vi "Frame Sample FIFO Experimental VI.vi"(8 "error in (no error)":errorcluster, 9 "reset in":bool, 10 "Hardware Configuration in":T1={"XY Stage"={"COM port"="", "XY stage available"=FALSE, "Baudrate"=0, "Type"=""}, "DAQ FPGA"={"Target"="RIO0", "input card type"=enum."AC Card", "Ref"=refnum, "Clock Freq (MHz) "=200.0, "Samples Wait after Trigger"=5080, "AOD fill"=4900, "StartupDelay"=0, "Slip Cycle (clock cycles)"=600000, "Add Cycle"=TRUE}, "Control system"={"Contrl Sys Available Ind"=FALSE, "Control system.FPGA Type"=enum."Virtex 7", "Control system.Network adapter name"="", "Control system.MAC address"="", "Control system.Ethernet Port"=0, "Ethernet opened"=FALSE, "Ctrl FPGA Clock (MHz)"=240.0, "AOD 1 Amplitude"=0, "AOD 2 Amplitude"=0, "AOD 3 Amplitude"=0, "AOD 4 Amplitude"=0, "AOD 5 Amplitude"=0, "AOD 6 Amplitude"=0, "Data Time Interval (ns)"=0.0, "T0 (ns)"=0.0, "Ta (ns)"=0.0}, "Encoder"={"IP address"="224.0.1.103", "Port"=7000, "Wheel radius (cm)"=16.0, "Encoder Trigger"=""}, "DAQmx Chan"={"Pockels AO"="", "Hard shutter AO"="", "PMT AOs"="", "Galvo AOs"="", "Power meter AI"=""}, "Computer MAC address"="", "Cam VidRec"={"DO flag-Video record"="", "DO flag-Trial start"=""}, "Externalise Triggers"=FALSE, "MC Supported"=FALSE, "Laser wavelength (nm)"=920.0} {"Laser wavelength (nm)" min=800.0 max=1080.0 step=1.0; "Encoder"."Wheel radius (cm)" format="%#_13g"; "Control system"."Control system.Ethernet Port" min=0 max=2048 step=1; "Control system"."Ctrl FPGA Clock (MHz)" min=80.0 max=500.0 step=1.0; "Control system"."Data Time Interval (ns)" min=0.0 max=2048.0 step=1.0; "Control system"."Ta (ns)" min=0.0 max=2048.0 step=1.0; "Control system"."T0 (ns)" min=0.0 max=2048.0 step=1.0; "Control system"."AOD 6 Amplitude" min=0 max=2048 step=1; "Control system"."AOD 5 Amplitude" min=0 max=2048 step=1; "Control system"."AOD 4 Amplitude" min=0 max=2048 step=1; "Control system"."AOD 3 Amplitude" min=0 max=2048 step=1; "Control system"."AOD 2 Amplitude" min=0 max=2048 step=1; "Control system"."AOD 1 Amplitude" min=0 max=2048 step=1}) -> (0 "error out":errorcluster, 1 "reset out":bool, 2 "Hardware Configuration out":T1={"XY Stage"={"COM port"="", "XY stage available"=FALSE, "Baudrate"=0, "Type"=""}, "DAQ FPGA"={"Target"="RIO0", "input card type"=enum."AC Card", "Ref"=refnum, "Clock Freq (MHz) "=200.0, "Samples Wait after Trigger"=5080, "AOD fill"=4900, "StartupDelay"=0, "Slip Cycle (clock cycles)"=600000, "Add Cycle"=TRUE}, "Control system"={"Contrl Sys Available Ind"=FALSE, "Control system.FPGA Type"=enum."Virtex 7", "Control system.Network adapter name"="", "Control system.MAC address"="", "Control system.Ethernet Port"=0, "Ethernet opened"=FALSE, "Ctrl FPGA Clock (MHz)"=240.0, "AOD 1 Amplitude"=0, "AOD 2 Amplitude"=0, "AOD 3 Amplitude"=0, "AOD 4 Amplitude"=0, "AOD 5 Amplitude"=0, "AOD 6 Amplitude"=0, "Data Time Interval (ns)"=0.0, "T0 (ns)"=0.0, "Ta (ns)"=0.0}, "Encoder"={"IP address"="224.0.1.103", "Port"=7000, "Wheel radius (cm)"=16.0, "Encoder Trigger"=""}, "DAQmx Chan"={"Pockels AO"="", "Hard shutter AO"="", "PMT AOs"="", "Galvo AOs"="", "Power meter AI"=""}, "Computer MAC address"="", "Cam VidRec"={"DO flag-Video record"="", "DO flag-Trial start"=""}, "Externalise Triggers"=FALSE, "MC Supported"=FALSE, "Laser wavelength (nm)"=920.0} {"Laser wavelength (nm)" min=800.0 max=1080.0 step=1.0; "Encoder"."Wheel radius (cm)" format="%#_13g"; "Control system"."Control system.Ethernet Port" min=0 max=2048 step=1; "Control system"."Ctrl FPGA Clock (MHz)" min=80.0 max=500.0 step=1.0; "Control system"."Data Time Interval (ns)" min=0.0 max=2048.0 step=1.0; "Control system"."Ta (ns)" min=0.0 max=2048.0 step=1.0; "Control system"."T0 (ns)" min=0.0 max=2048.0 step=1.0; "Control system"."AOD 6 Amplitude" min=0 max=2048 step=1; "Control system"."AOD 5 Amplitude" min=0 max=2048 step=1; "Control system"."AOD 4 Amplitude" min=0 max=2048 step=1; "Control system"."AOD 3 Amplitude" min=0 max=2048 step=1; "Control system"."AOD 2 Amplitude" min=0 max=2048 step=1; "Control system"."AOD 1 Amplitude" min=0 max=2048 step=1}, 3 "tdms file out":refnum<k34>)   [LabVIEW 2020]
uses:
  <vilib>/rvi/interface/nirviMethod/nirviMethod.xnode
  <vilib>/rvi/errors/niLvFpgaMergeErrorWithErrorCode.vi
  <vilib>/FPGAPlugInAG/Dynamic/niLvFpga_ReadFifo_Dynamic.vi
  RIG-SPECIFIC FILES/FPGA Refs/FPGA Ref.ctl
  Typedefs/Sys Configuration.ctl
  <vilib>/userDefined/High Color/nirio_resource_hc.ctl
  Typedefs/DAQ FPGA config cluster.ctl
  Typedefs/DAQmx physical channels cluster.ctl
  Typedefs/CTRL system config cluster.ctl
  Typedefs/XY Stage config cluster.ctl
  Typedefs/FPGA input type AC-DC.ctl
  Typedefs/Encoder config cluster.ctl
  Typedefs/Cam VidRec HW config setup cluster.ctl
panel:
  out "Numeric":u16
  in  "Loop iteration time (ms)":u32
  out "Loop iteration time (ms)":u32
  out "largest # of points returned in a single read":u32
  out "[I16] Data Array":i16[](array[numeric])
  out "Number of points":i32
  in  "TDMS file base path":path=path "C:/Users/SilverLab/Desktop/Grabbed Single Frame Data"
  out "[I16] Data Graph":i16[](graph)
  # "NOT CURRENTLY IN USE"
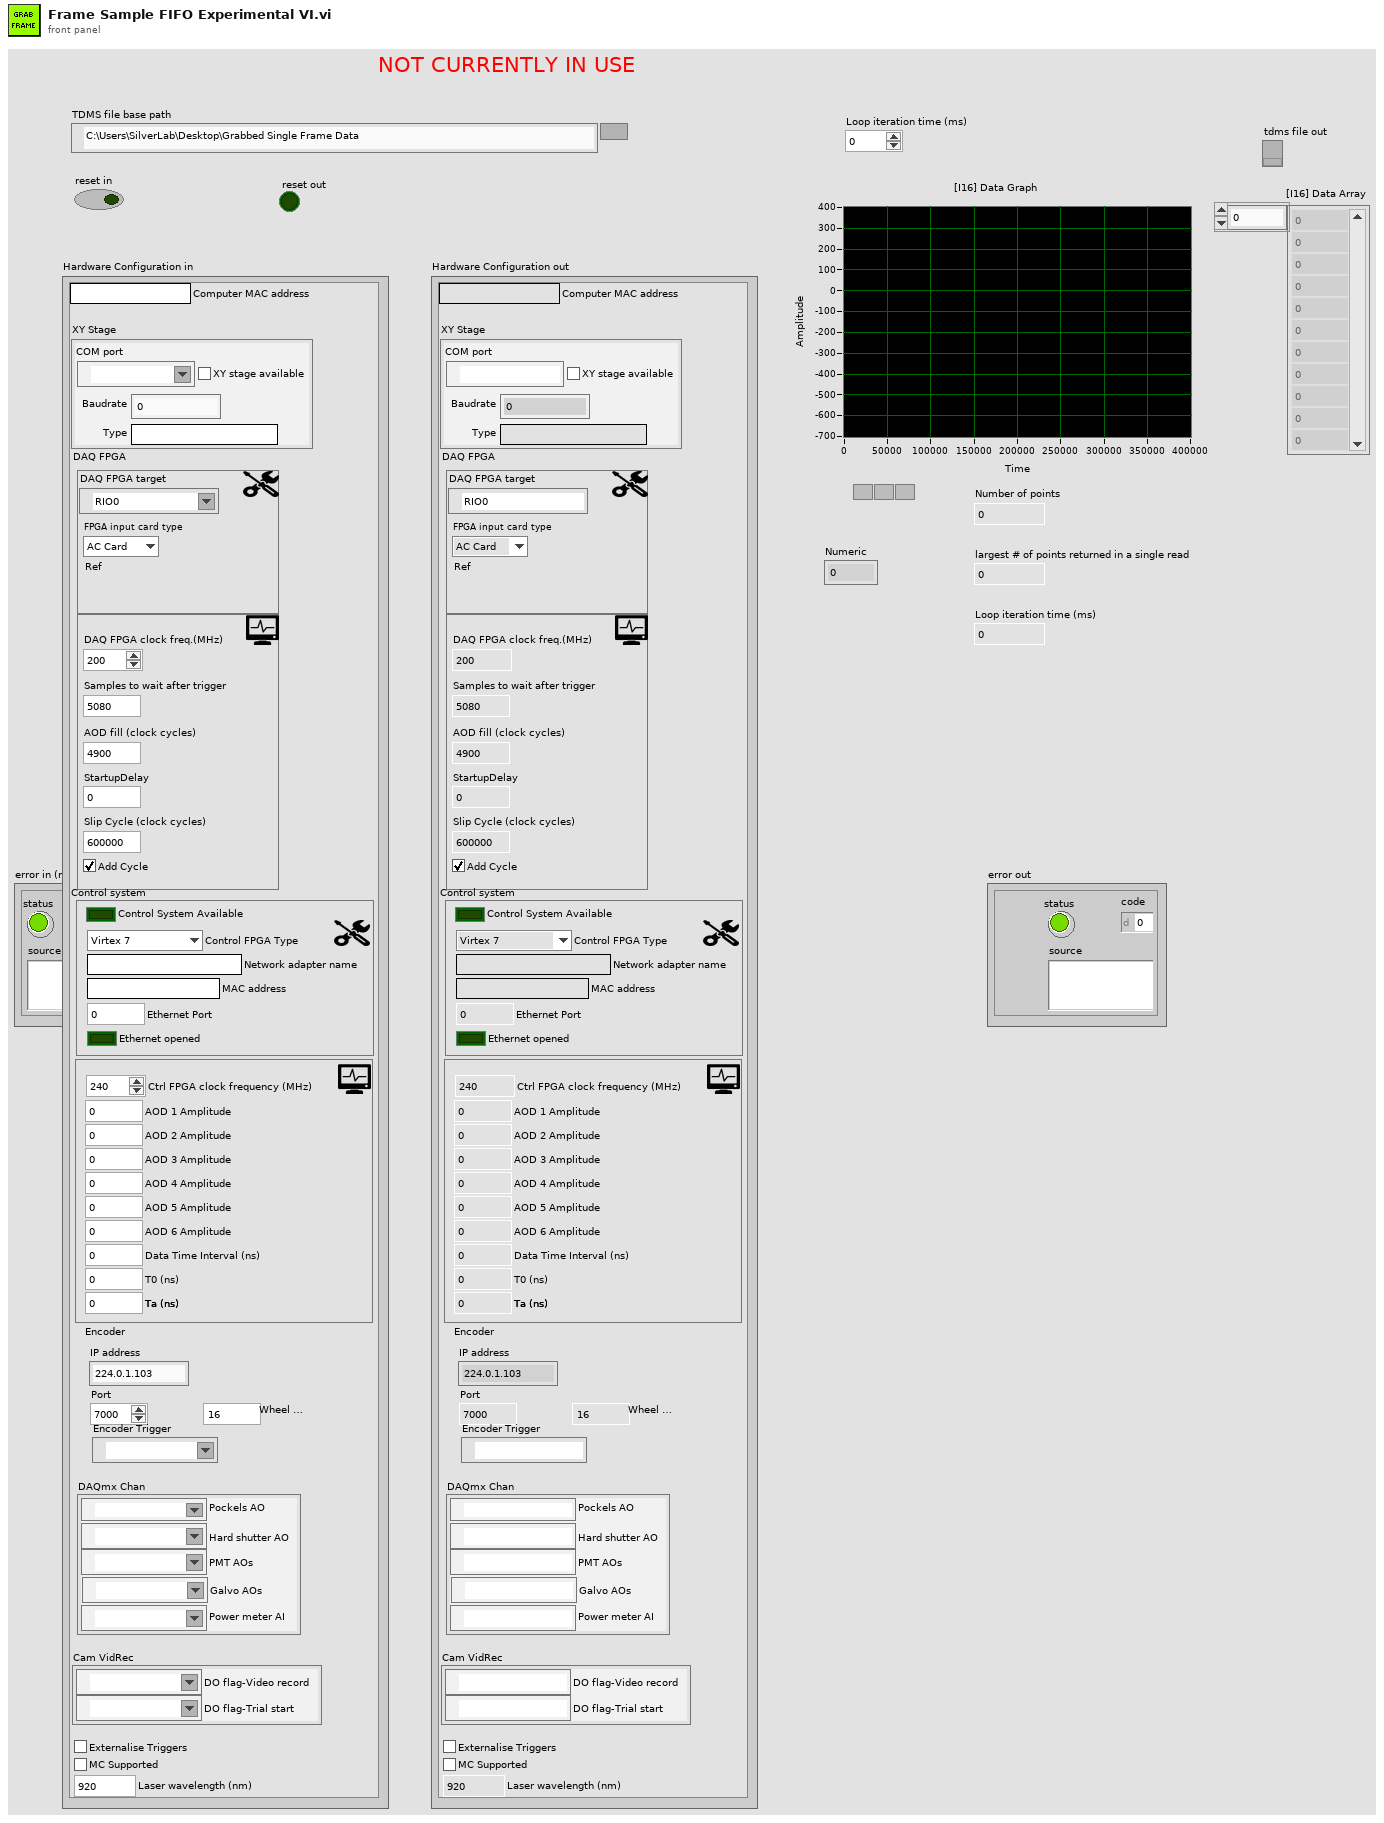
[diagram p1: front panel]
types:
  T1 = typedef "Sys Configuration.ctl" = cluster{"XY Stage":T2, "DAQ FPGA":T3, "Control system":T7, "Encoder":T8, "DAQmx Chan":T9, "Computer MAC address":string, "Cam VidRec":T10, "Externalise Triggers":bool, "MC Supported":bool, "Laser wavelength (nm)":dbl}
  T2 = typedef "XY Stage config cluster.ctl" = cluster{"COM port":refnum<visa-resource-name>, "XY stage available":bool, "Baudrate":i32, "Type":string}
  T3 = typedef "DAQ FPGA config cluster.ctl" = cluster{"Target":T4, "input card type":T5, "Ref":T6, "Clock Freq (MHz) ":dbl, "Samples Wait after Trigger":u16, "AOD fill":u16, "StartupDelay":i32, "Slip Cycle (clock cycles)":u32, "Add Cycle":bool}
  T4 = typedef "nirio_resource_hc.ctl" = tag
  T5 = typedef "FPGA input type AC-DC.ctl" = enum16{"AC Card", "DC Card"}
  T6 = typedef "FPGA Ref.ctl" = refnum<k20>
  T7 = typedef "CTRL system config cluster.ctl" = cluster{"Contrl Sys Available Ind":bool, "Control system.FPGA Type":enum16{"Virtex 5", "Virtex 7"}, "Control system.Network adapter name":string, "Control system.MAC address":string, "Control system.Ethernet Port":i16, "Ethernet opened":bool, "Ctrl FPGA Clock (MHz)":dbl, "AOD 1 Amplitude":i16, "AOD 2 Amplitude":i16, "AOD 3 Amplitude":i16, "AOD 4 Amplitude":i16, "AOD 5 Amplitude":i16, "AOD 6 Amplitude":i16, "Data Time Interval (ns)":dbl, "T0 (ns)":dbl, "Ta (ns)":dbl}
  T8 = typedef "Encoder config cluster.ctl" = cluster{"IP address":string, "Port":u16, "Wheel radius (cm)":dbl, "Encoder Trigger":tag}
  T9 = typedef "DAQmx physical channels cluster.ctl" = cluster{"Pockels AO":tag, "Hard shutter AO":tag, "PMT AOs":tag, "Galvo AOs":tag, "Power meter AI":tag}
  T10 = typedef "Cam VidRec HW config setup cluster.ctl" = cluster{"DO flag-Video record":tag, "DO flag-Trial start":tag}
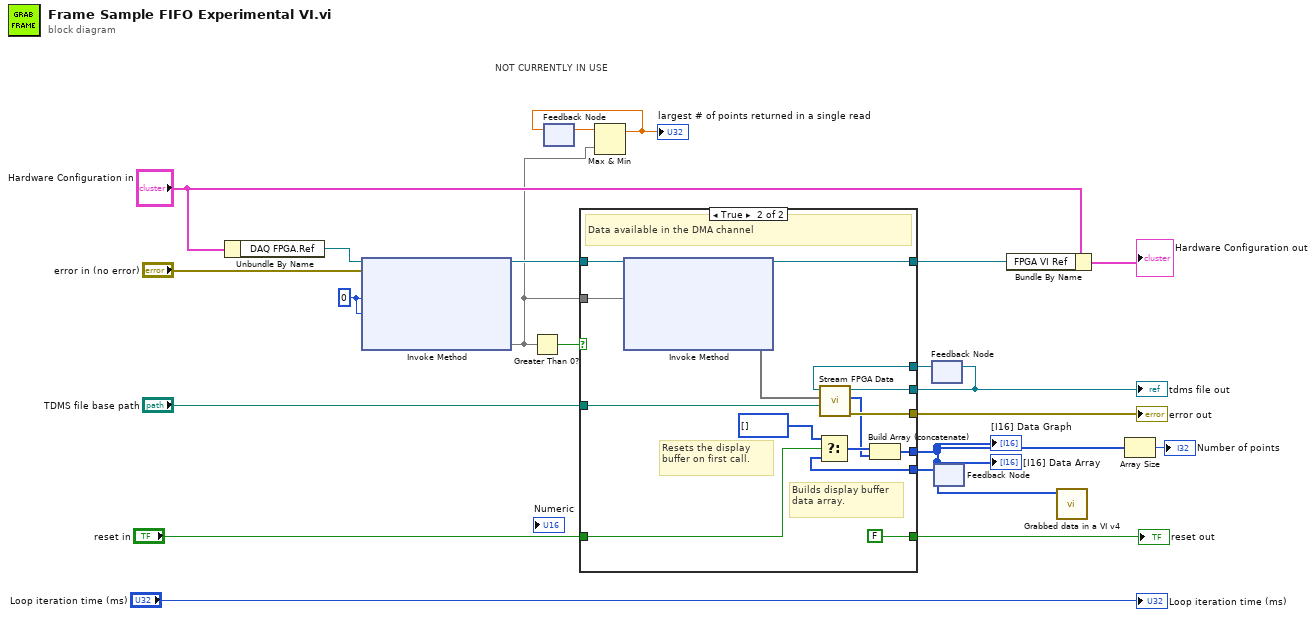
[diagram p0: block diagram]
diagram:
  w15 = 0 ("Timeout (ms)")
  # "NOT CURRENTLY IN USE"
  n1 = Unbundle By Name("Hardware Configuration in") -> ("DAQ FPGA.Ref"=w21:T6)
  n2 = xnode ("Invoke Method")("FPGA VI Reference In"=w21, "error in"="error in (no error)", "Number of Elements"=w15, "Timeout (ms)"=w15) -> ("FPGA VI Reference Out"=w11:T6, "Elements Remaining"=w4)  [unwired: 2 out]
  n3 = Greater Than 0?(x=w4) -> (x > 0?=w12:bool)
  n4 = feedback #1() -> (w5:dbl)  [unwired: 1 in]
  n5 = Max & Min(x=w5, y=w4) -> (max(x,y)=w3:dbl)  [unwired: 1 out]
  "largest # of points returned in a single read" <- w3
  n6 = feedback-in #1(w3) -> ()
  n7 = feedback #2() -> (w17:refnum<k34>)  [unwired: 1 in]
  n8 = feedback #3() -> (w16:i16[])  [unwired: 1 in]
  n9 = case shown="True" w12 {
    tunnel: [_ w40] -> w19
    tunnel: [w25 w39] -> w9
    tunnel: "TDMS file base path" -> [_ w38]
    tunnel: [w24 w36] -> w1
    tunnel: w17 -> [w25 w32]
    tunnel: w16 -> [w24 w31]
    tunnel: [w23 w30] -> w10
    tunnel: w4 -> [_ w29]
    tunnel: w11 -> [w23 w28]
    tunnel: "reset in" -> [w22 w27]
    tunnel: [w22 FALSE] -> w7
    frame False {
      # "No data available on the DMA channel"
    }
    frame True {
      # "Builds display buffer data array."
      # "Resets the display buffer on first call."
      # "Data available in the DMA channel"
      n10 = xnode "Invoke Method"("FPGA VI Reference In"=w28, "Number of Elements"=w29) -> ("FPGA VI Reference Out"=w30:T6, "Data"=w37:void[])  [unwired: 2 in, 2 out]
      n11 = Select(t=i16[] [], s=w27, f=w31) -> (s? t:f=w34:i16[])
      n12 = call "Stream FPGA Data.vi"("TDMS file base path"=w38, "DMA Data Values"=w37, "tdms file in"=w32) -> ("error out"=w40:errorcluster, "[I16] All points in correct chronological order"=w33:i16[], "tdms file out"=w39:refnum<k34>)  [unwired: 6 in]
      n13 = Build Array (concatenate)(w34, w33) -> (w36:i16[])
    }
  }
  "[I16] Data Graph" <- w1
  "[I16] Data Array" <- w1
  "tdms file out" <- w9
  "error out" <- w19
  "reset out" <- w7
  n14 = feedback-in #2(w9) -> ()
  n15 = feedback-in #3(w1) -> ()
  n16 = Bundle By Name(cluster="Hardware Configuration in", "FPGA VI Ref"=w10) -> (→"Hardware Configuration out":T1)
  n17 = call "Grabbed data in a VI v4.vi"("[I16] Source Graph\n(samples added to reach 320000)"=w1) -> ()  [unwired: 11 in]
  n18 = Array Size(array=w1) -> (size(s)=→"Number of points":i32)
  "Loop iteration time (ms)" <- "Loop iteration time (ms)"
